vi "PH_ImageOperator.evt call set Energy Settings.vi"(0 "i ref in":refnum<vi>, 1 "Instance":string, 2 "Calculate":bool, 3 "expected value [mJ]":dbl, 4 "Tolerance [%]":dbl, 5 "error in (no error)":errorcluster) -> (14 "i ref out":refnum<vi>, 19 "error out":errorcluster)   [LabVIEW 2014, in "PH_ImageOperator.lvlib"]
doc: "This VI calls the event case \"SetEnergySettings\" by a simple call."
uses:
  PH_ImageOperator.lvlib
  CS_Core/CSSystem/CoreLib/CoreLib.double 2 byte array.vi
  CS_Core/CSSystem/CoreLib/CoreLib.short 2 byte array.vi
  CS_Core/CSSystem/CoreLib/CoreLib.lvlib
  CS_Core/BaseProcess/BaseProcess.lvlib
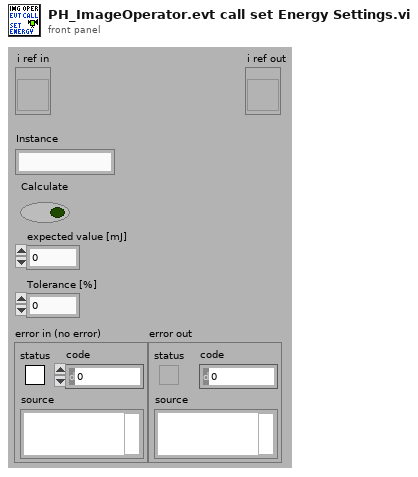
[diagram p1: front panel]
types:
  T1 = typedef "CoreDefs.rawDataType.ctl" = i8[]
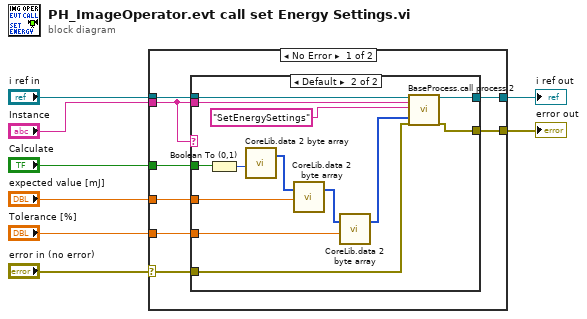
[diagram p0: block diagram]
diagram:
  n1 = case shown="No Error" "error in (no error)" {
    selector: "error in (no error)" -> [w12 w32]
    tunnel: [w16 w33] -> w7
    tunnel: [w15 w32] -> w6
    tunnel: "i ref in" -> [w14 w33]
    tunnel: "Instance" -> [w11 _]
    tunnel: "Calculate" -> [w13 _]
    tunnel: "expected value [mJ]" -> [w10 _]
    tunnel: "Tolerance [%]" -> [w9 _]
    frame No Error {
      n2 = case shown="Default" w11 {
        tunnel: [w18 w30] -> w16
        tunnel: [w17 w29] -> w15
        tunnel: w14 -> [w18 w28]
        tunnel: w11 -> [_ w27]
        tunnel: w13 -> [_ w25]
        tunnel: w12 -> [w17 w24]
        tunnel: w10 -> [_ w20]
        tunnel: w9 -> [_ w19]
        frame "N/A" {
        }
        frame Default {
          n3 = Boolean To (0,1)(Boolean=w25) -> (0, 1=w26:i16)
          n4 = call-poly "CoreLib.data 2 byte array.vi"("i16"=w26) -> ("byteArray out"=w23:T1)  [unwired: 18 in]
          n5 = call-poly "CoreLib.data 2 byte array.vi"("byteArray"=w23, "f64"=w20) -> ("byteArray out"=w22:T1)  [unwired: 17 in]
          n6 = call-poly "CoreLib.data 2 byte array.vi"("byteArray"=w22, "f64"=w19) -> ("byteArray out"=w21:T1)  [unwired: 17 in]
          n7 = call "BaseProcess.call process 2.vi"("i ref in"=w28, "Object"=w27, "Selector"="SetEnergySettings", "Data"=w21, "error in (no error)"=w24) -> ("i ref out"=w30:refnum<vi>, "error out"=w29:errorcluster)  [unwired: 13 in]
        }
      }
    }
    frame Error {
    }
  }
  "i ref out" <- w7
  "error out" <- w6
